vi "RobotState_fromDrive_get.vi"(8 "error in (no error)":errorcluster) -> (0 "error out":errorcluster, 2 "RobotState_fromDrive":T1)   [LabVIEW 2009, in "NetworkVarTarget.lvlib"]
uses:
  NetworkVarTarget.lvlib
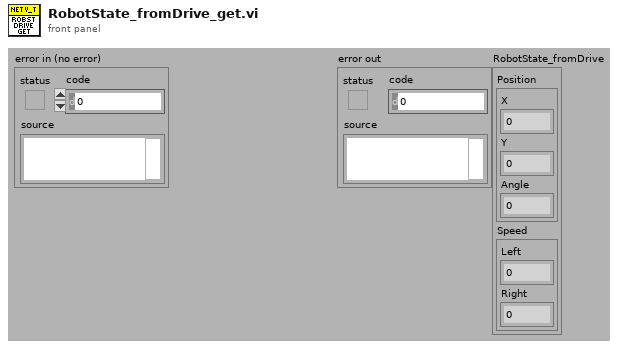
[diagram p1: front panel]
types:
  T1 = cluster{"Position":cluster{"X":dbl, "Y":dbl, "Angle":dbl}, "Speed":cluster{"Left":dbl, "Right":dbl}}
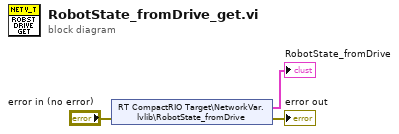
[diagram p0: block diagram]
diagram:
  n1 = shared-variable "RT CompactRIO Target\\NetworkVar.lvlib\\RobotState_fromDrive"(error in="error in (no error)") -> (→"RobotState_fromDrive":T1, error out=→"error out":errorcluster)
